vi "commit VI reference.vi"(8 "error in":errorcluster, 10 "VI Refnum in":refnum<vi>, 11 "UI Reference configuration in":refnum<class "UI Reference configuration.lvclass">) -> (0 "error out":errorcluster, 2 "VI Refnum out":refnum<vi>, 3 "UI Reference configuration out":refnum<class "UI Reference configuration.lvclass">)   [LabVIEW 2015, in "UI Reference configuration.lvclass"]
uses:
  UI Reference configuration.lvclass
  UI Reference configuration.lvclass/UI Reference configuration.ctl
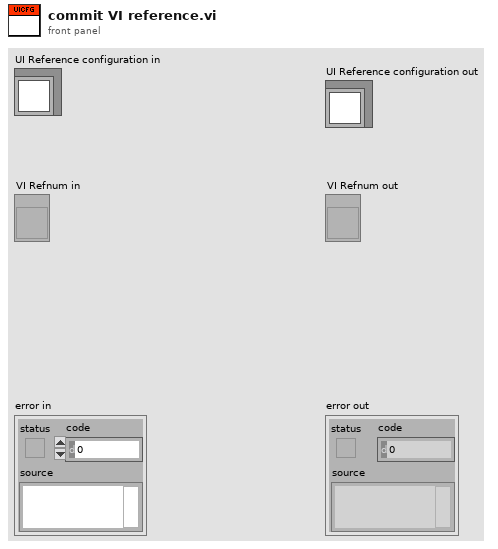
[diagram p1: front panel]
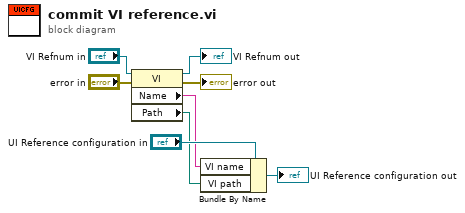
[diagram p0: block diagram]
diagram:
  n1 = property class="VI"(reference="VI Refnum in", error in="error in") -> (reference out=→"VI Refnum out":refnum<vi>, error out=→"error out":errorcluster, "Name"=w3:string, "Path"=w2:path)
  n2 = Bundle By Name(cluster="UI Reference configuration in", "VI name"=w3, "VI path"=w2) -> (→"UI Reference configuration out":refnum<class "UI Reference configuration.lvclass">)
